vi "ex4_moje.vi"() -> ()   [LabVIEW 2022 SP3]
panel:
  in  "stop":bool
  in  "User":string
  in  "ok button":bool
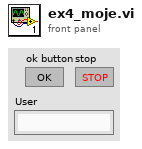
[diagram p1: front panel]
types:
  T1 = enum16{"open", "replace", "create", "open or create", "replace or create", "replace or create with confirmation"}
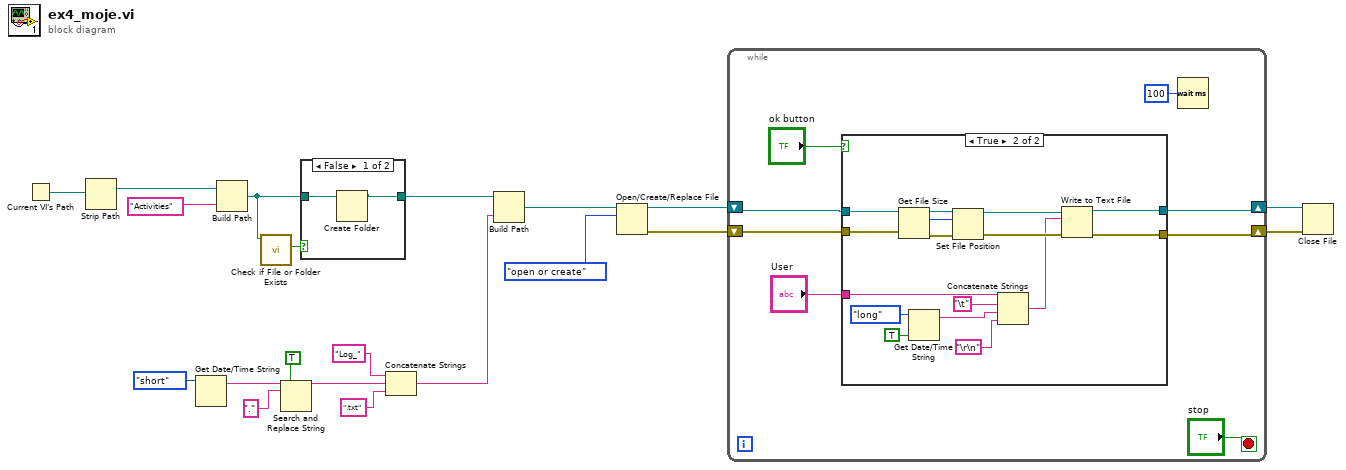
[diagram p0: block diagram]
diagram:
  n1 = Current VI's Path() -> (path=w20:path)
  n2 = Strip Path(path=w20) -> (stripped path=w19:path)  [unwired: 1 out]
  n3 = Get Date/Time String(date format (0)=enum16{"short", "long", "abbreviated"}."short") -> (date string=w14:string)  [unwired: 2 in, 1 out]
  n4 = Build Path(base path=w19, name or relative path="Activities") -> (appended path=w1:path)
  n5 = call <vilib>:"Check if File or Folder Exists.vi"("path"=w1) -> ("file or folder exists?"=w2:bool)  [unwired: 8 in, 2 out]
  n6 = Search and Replace String(replace all?=TRUE ("replace all? (F)"), input string=w14, search string=".") -> (result string=w11:string)  [unwired: 5 in, 3 out]
  n7 = case shown="False" w2 {
    tunnel: w1 -> [w22 w23]
    tunnel: [w21 w23] -> w17
    frame False {
      n8 = Create Folder(path (use dialog)=w22) -> (created path=w21:path)  [unwired: 2 in, 2 out]
    }
    frame True {
    }
  }
  n9 = Concatenate Strings("Log_" ("string"), w11, ".txt" ("string")) -> (w9:string)
  n10 = Build Path(base path=w17, name or relative path=w9) -> (appended path=w8:path)
  n11 = Open/Create/Replace File(file path (use dialog)=w8, operation (0:open)=T1."open or create") -> (refnum out=w6:refnum<file>, error out=w5:errorcluster)  [unwired: 4 in, 1 out]
  n12 = while {
    shift-right: [w26] -> w4
    shift-left: w6 -> [w29]
    shift-right: [w25] -> w3
    shift-left: w5 -> [w28]
    stop <- "stop" stop-if-true
    n13 = case shown="True" "ok button" {
      tunnel: w29 -> [w33 w49]
      tunnel: w28 -> [w32 w48]
      tunnel: "User" -> [_ w44]
      tunnel: [w33 w35] -> w26
      tunnel: [w32 w34] -> w25
      frame False {
      }
      frame True {
        n14 = Get File Size(file=w49, error in=w48) -> (refnum out=w47:refnum<file>, size (in bytes)=w46:i64, 0:w45:errorcluster)
        n15 = Get Date/Time String(date format (0)=enum16{"short", "long", "abbreviated"}."long", want seconds? (F)=TRUE) -> (date string=w40:string)  [unwired: 1 in, 1 out]
        n16 = Set File Position(offset (in bytes) (0)=w46, refnum=w47, error in=w45) -> (refnum out=w38:refnum<file>, error out=w37:errorcluster)  [unwired: 1 in]
        n17 = Concatenate Strings(w44, "\t", w40, "\r\n") -> (w36:string)
        n18 = Write to Text File(file (use dialog)=w38, text=w36, error in=w37) -> (refnum out=w35:refnum<file>, error out=w34:errorcluster)  [unwired: 1 in, 1 out]
      }
    }
    n19 = Wait (ms)(milliseconds to wait=u32 100) -> ()  [unwired: 1 out]
  }
  n20 = Close File(refnum=w4, error in=w3) -> ()  [unwired: 2 out]
